vi "Signal Measurement Complete.vi"(8 "error in (no error)":errorcluster) -> (0 "error out":errorcluster, 5 "done channel":T1)   [LabVIEW 2025, in "auto-vision-plugin.lvclass"]
doc: "Signal the loop that monitors for cancellation that the measurement has completed normally and that the loop should exit."
uses:
  auto-vision-plugin.lvclass
  <extravilib>/ChannelInstances/Event Messenger-bool/))Channel.ctl
  <extravilib>/ChannelInstances/Event Messenger-bool/))Channel.vi
  auto-vision-plugin.lvclass/auto-vision-plugin.ctl
  <extravilib>/ChannelInstances/Event Messenger-bool.lvlib
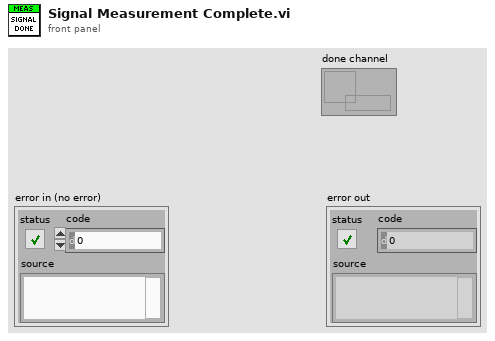
[diagram p1: front panel]
types:
  T1 = typedef "Event Messenger-bool.lvlib/))Channel.ctl" = refnum<queue>
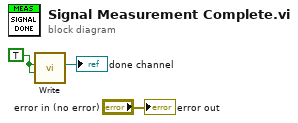
[diagram p0: block diagram]
diagram:
  w2 = TRUE
  n1 = call <extravilib>:"Write.vi"("last element? (F)"=w2, "element"=w2) -> ("channel"=→"done channel":T1)  [unwired: 8 in, 1 out]
  "error out" <- "error in (no error)"
